vi "Teardown Device.vi"(4 "error in (no error)":errorcluster) -> (0 "error out":errorcluster, 2 "function return":i32)   [LabVIEW 2020, in "MPH16.lvlib"]
doc: "long TeardownDevice();"
uses:
  MPH16.lvlib
  ThorPinholeStepper.dll
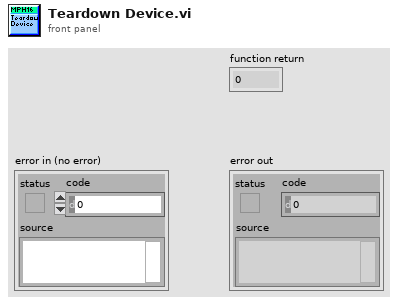
[diagram p1: front panel]
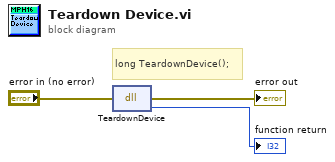
[diagram p0: block diagram]
diagram:
  # "long TeardownDevice();"
  n1 = dll-call lib="D:/software/TweezerTron Project/Instruments/Thorlabs/MPH_SDK/ThorPinholeStepper.*" fn="TeardownDevice"(error in="error in (no error)") -> (error out=→"error out":errorcluster, →"function return":i32)  [unwired: 2 in, 1 out]
